vi "Get Config Properties.vi"(8 "error in (no error)":errorcluster, 11 "LatestValueCalculation in":refnum<class "LatestValueCalculation.lvclass">) -> (0 "error out":errorcluster, 3 "LatestValueCalculation out":refnum<class "LatestValueCalculation.lvclass">)   [LabVIEW 2015, in "LatestValueCalculation.lvclass"]
uses:
  LatestValueCalculation.lvclass
  WaveformCalculation/WaveformCalculation.lvclass
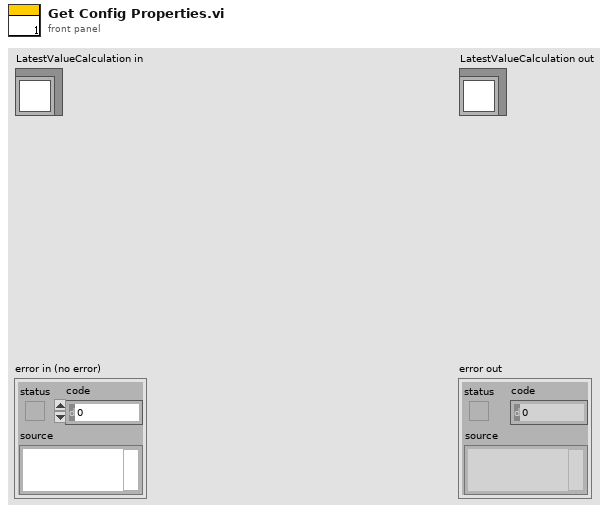
[diagram p1: front panel]
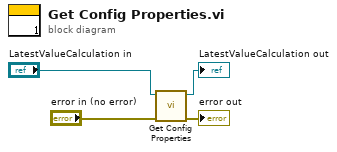
[diagram p0: block diagram]
diagram:
  n1 = call-parent "Get Config Properties.vi"("error in (no error)"="error in (no error)", "WaveformCalculation in"="LatestValueCalculation in") -> ("error out"=→"error out":errorcluster, "WaveformCalculation out"=→"LatestValueCalculation out":refnum<class "LatestValueCalculation.lvclass">)  [unwired: 8 in]
